vi "Google Earth - Version info.vi"(8 "error in":errorcluster, 11 "Refnum In":refnum<k7>) -> (0 "error out":errorcluster, 2 "Version":string, 3 "Refnum Out":refnum<k7>, 5 "VersionAppType":i32(ring) items=["EnterpriseClientGE"=0, "ProGE"=1, "PlusGE"=2, "FreeGE"=5, "UnknownGE"=255])   [LabVIEW 2011]
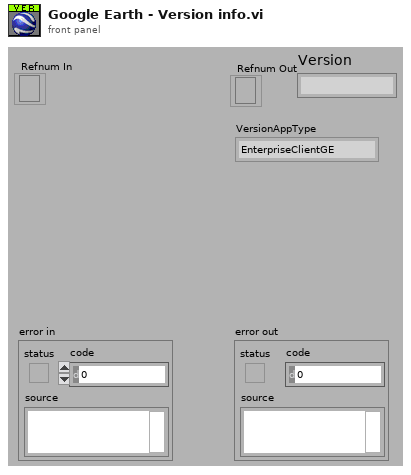
[diagram p1: front panel]
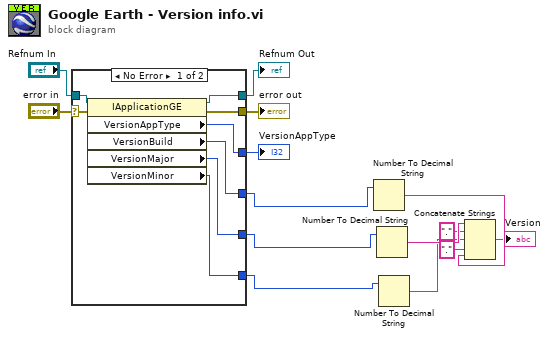
[diagram p0: block diagram]
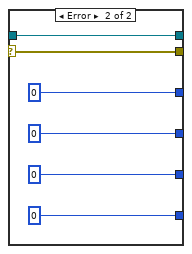
[diagram p2: hidden frame]
diagram:
  n1 = case shown="No Error" "error in" {
    selector: "error in" -> [w15 w28]
    tunnel: [w22 w28] -> w14
    tunnel: [w21 w27] -> w13
    tunnel: [w20 0 ("VersionMinor")] -> w7
    tunnel: [w19 0 ("VersionMajor")] -> w8
    tunnel: [w18 0 ("VersionBuild")] -> w9
    tunnel: [w17 0 ("VersionAppType")] -> w10
    tunnel: "Refnum In" -> [w16 w27]
    frame No Error {
      n2 = property class="IApplicationGE"(reference=w16, error in=w15) -> (reference out=w21:refnum<k7>, error out=w22:errorcluster, "VersionAppType"=w17:i32, "VersionBuild"=w18:i32, "VersionMajor"=w19:i32, "VersionMinor"=w20:i32)
    }
    frame Error {
    }
  }
  "VersionAppType" <- w10
  "error out" <- w14
  "Refnum Out" <- w13
  n3 = Number To Decimal String(number=w9) -> (decimal integer string=w2:string)  [unwired: 1 in]
  n4 = Number To Decimal String(number=w8) -> (decimal integer string=w6:string)  [unwired: 1 in]
  n5 = Number To Decimal String(number=w7) -> (decimal integer string=w4:string)  [unwired: 1 in]
  n6 = Concatenate Strings(w6, "." ("string"), w4, "." ("string"), w2) -> (→"Version":string)
